vi "Write to Hardware.vi"(8 "error in":errorcluster, 9 "Trigger Values":dbl[](array[numeric]), 10 "Values in":dbl[](array[numeric]), 11 "Address Based Execution Unit Implementation in":refnum<class "Tx Acyclic Execution Unit.lvclass">) -> (0 "error out":errorcluster, 1 "Trigger Values out":dbl[](array[numeric]), 2 "Values out":dbl[](array[numeric]), 3 "Address Based Execution Unit Implementation out":refnum<class "Tx Acyclic Execution Unit.lvclass">)   [LabVIEW 2020, in "AIM MIL-STD-1553 Engine.lvlib" / "Implementation.lvlib" / "Tx Acyclic Execution Unit.lvclass"]
uses:
  Tx Acyclic Execution Unit.lvclass
  Tx Acyclic Execution Unit.lvclass/Tx Acyclic Execution Unit.ctl
  <instrlib>/BTI1553Lib/BTI1553LV.lvlib
  <instrlib>/BTI1553Lib/Private/BC/Data/BC Transmit Acyclic Frame.vi
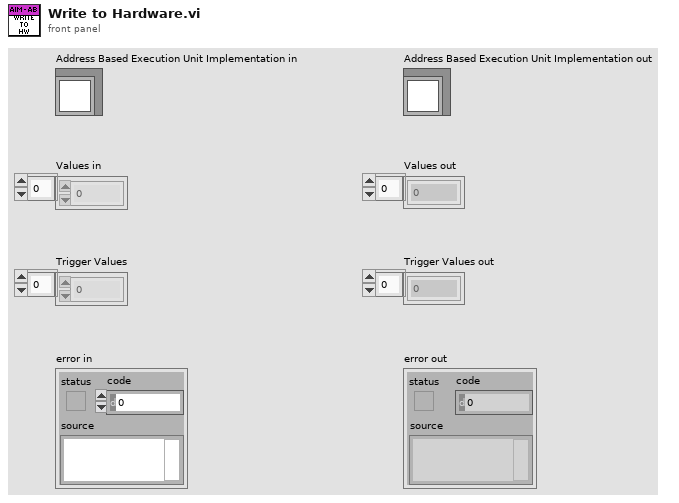
[diagram p1: front panel]
types:
  T1 = typedef "AIM MIL-STD-1553 Engine.lvlib/Implementation.lvlib/Address Based Execution Unit.lvclass/Acyclic Trigger Info.ctl" = cluster{"bus controller handle":u64, "name":string}
  T2 = typedef "AIM MIL-STD-1553 Engine.lvlib/Implementation.lvlib/Address Based Execution Unit.lvclass/Address Write Info.ctl" = cluster{"terminal address":T3, "terminal handle":u64}
  T3 = typedef "Address.ctl" = u16
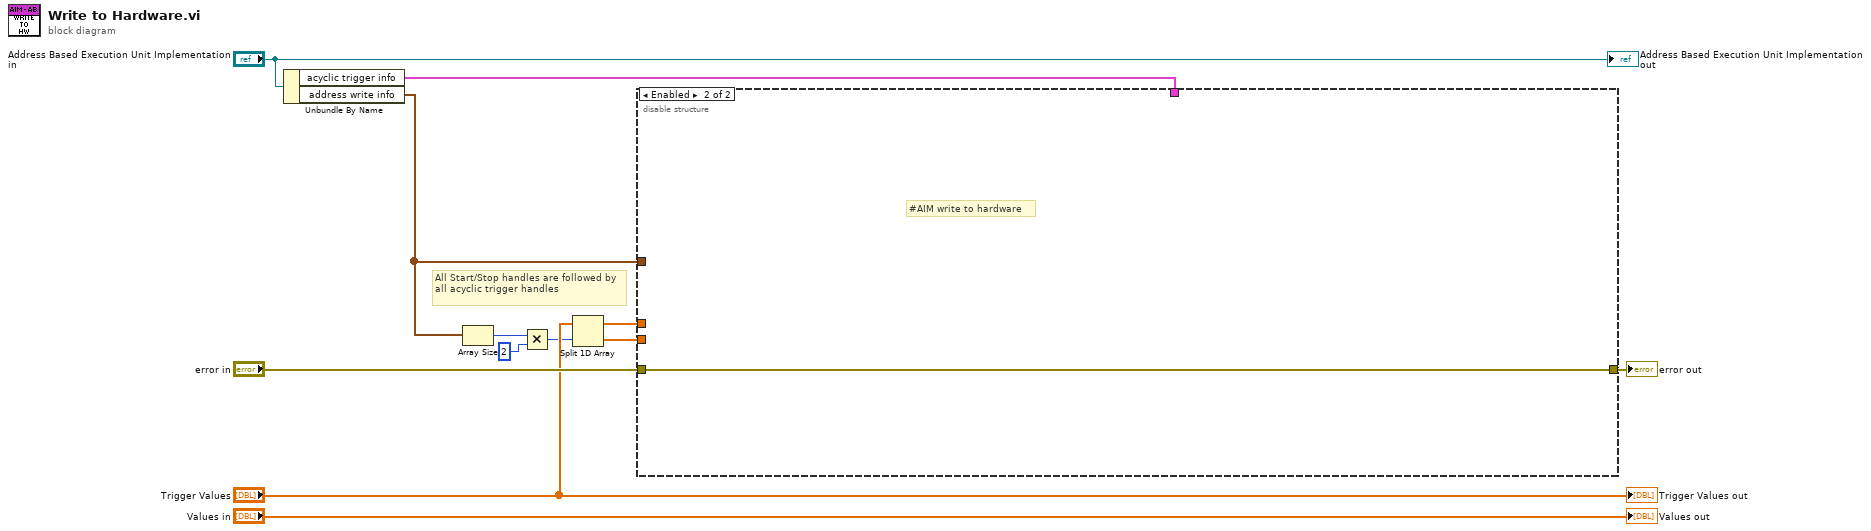
[diagram p0: block diagram]
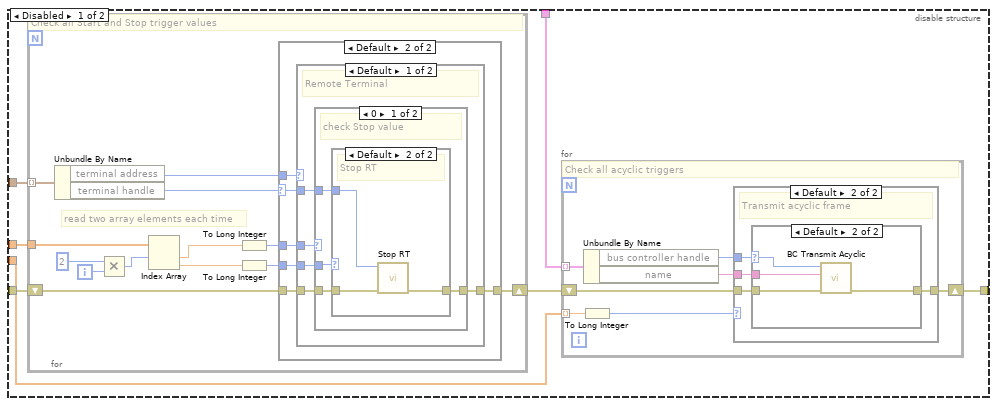
[diagram p2: hidden frame]
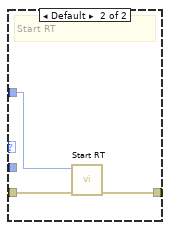
[diagram p7: hidden frame]
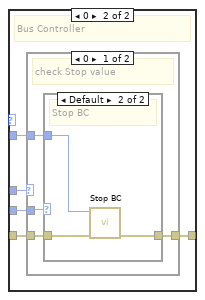
[diagram p8: hidden frame]
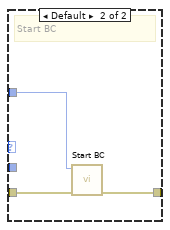
[diagram p10: hidden frame]
diagram:
  # "All Start/Stop handles are followed by all acyclic trigger handles"
  n1 = Unbundle By Name("Address Based Execution Unit Implementation in") -> ("acyclic trigger info"=w1:T1[], "address write info"=w8:T2[])
  n2 = Array Size(array=w8) -> (size(s)=w7:i32)
  n3 = Multiply(x=w7, y=2) -> (x*y=w5:i32)
  n4 = Split 1D Array(array="Trigger Values", index=w5) -> (first subarray=w9:dbl[], second subarray=w2:dbl[])
  n5 = disable-structure shown="Enabled" {
    disable-tunnel: "error in" -> [w19 w89]
    disable-tunnel: w9 -> [w18 _]
    disable-tunnel: w8 -> [w17 _]
    disable-tunnel: [w15 w89] -> w4
    disable-tunnel: w2 -> [w14 _]
    disable-tunnel: w1 -> [w13 _]
    frame Disabled {
      n6 = for {
        tunnel: w17 -> [w49] mode=indexing
        shift-right: [w44] -> w16
        shift-left: w19 -> [w45]
        tunnel: w18 -> [w47]
        i -> [w40]
        # "read two array elements each time"
        # "Check all Start and Stop trigger values"
        n7 = Unbundle By Name(w49) -> ("terminal address"=w48:T3, "terminal handle"=w46:u64)
        n8 = Multiply(x=2, y=w40) -> (x*y=w39:i32)
        n9 = Index Array(array=w47, index #1=w39) -> (element #1=w42:dbl, element #2=w43:dbl)  [unwired: 1 in]
        n10 = To Long Integer(number=w42) -> (32bit integer=w38:i32)
        n11 = To Long Integer(number=w43) -> (32bit integer=w37:i32)
        n12 = case shown="Default" w46 {
          selector: w46 -> [_ w55]
          tunnel: w48 -> [_ w56]
          tunnel: w45 -> [w50 w54]
          tunnel: [w50 w53] -> w44
          tunnel: w38 -> [_ w52]
          tunnel: w37 -> [_ w51]
          frame 0, -1 {
          }
          frame Default {
            n13 = case shown="Default" w56 {
              tunnel: w52 -> [w61 w77]
              tunnel: w51 -> [w57 w73]
              tunnel: w55 -> [w60 w76]
              tunnel: w54 -> [w59 w75]
              tunnel: [w58 w74] -> w53
              frame Default {
                # "Remote Terminal"
                n14 = case shown="0" w61 {
                  tunnel: w60 -> [w63 w71]
                  tunnel: w59 -> [w64 w72]
                  tunnel: [w62 w70] -> w58
                  tunnel: w57 -> [w65 _]
                  frame 0 {
                    # "check Stop value"
                    n15 = case shown="Default" w65 {
                      tunnel: w64 -> [w66 w69]
                      tunnel: w63 -> [_ w68]
                      tunnel: [w66 w67] -> w62
                      frame 0 {
                        # "do nothing"
                      }
                      frame Default {
                        # "Stop RT"
                        n16 = call <instrlib>:"Stop RT.vi"("error in (no error)"=w69, "remote terminal handle in"=w68) -> ("error out"=w67:errorcluster)  [unwired: 8 in, 1 out]
                      }
                    }
                  }
                  frame Default {
                    # "Start RT"
                    n17 = call <instrlib>:"Start RT.vi"("error in (no error)"=w72, "remote terminal handle in"=w71) -> ("error out"=w70:errorcluster)  [unwired: 8 in, 1 out]
                  }
                }
              }
              frame 0 {
                # "Bus Controller"
                n18 = case shown="0" w77 {
                  tunnel: w76 -> [w79 w86]
                  tunnel: w75 -> [w80 w88]
                  tunnel: [w78 w87] -> w74
                  tunnel: w73 -> [w81 _]
                  frame 0 {
                    # "check Stop value"
                    n19 = case shown="Default" w81 {
                      tunnel: w80 -> [w82 w85]
                      tunnel: w79 -> [_ w83]
                      tunnel: [w82 w84] -> w78
                      frame 0 {
                        # "do nothing"
                      }
                      frame Default {
                        # "Stop BC"
                        n20 = call <instrlib>:"Stop BC.vi"("error in (no error)"=w85, "bus controller handle in"=w83) -> ("error out"=w84:errorcluster)  [unwired: 8 in, 1 out]
                      }
                    }
                  }
                  frame Default {
                    # "Start BC"
                    n21 = call <instrlib>:"Start BC.vi"("error in (no error)"=w88, "bus controller handle in"=w86) -> ("error out"=w87:errorcluster)  [unwired: 8 in, 1 out]
                  }
                }
              }
            }
          }
        }
      }
      n22 = for {
        shift-right: [w25] -> w15
        shift-left: w16 -> [w26]
        tunnel: w13 -> [w22] mode=indexing
        tunnel: w14 -> [w24] mode=indexing
        # "Check all acyclic triggers"
        n23 = To Long Integer(number=w24) -> (32bit integer=w23:i32)
        n24 = Unbundle By Name(w22) -> ("bus controller handle"=w21:u64, "name"=w20:string)
        n25 = case shown="Default" w23 {
          tunnel: w26 -> [w27 w30]
          tunnel: [w27 w31] -> w25
          tunnel: w21 -> [_ w29]
          tunnel: w20 -> [_ w28]
          frame 0 {
            # "Do nothing"
          }
          frame Default {
            # "Transmit acyclic frame"
            n26 = case shown="Default" w29 {
              selector: w29 -> [_ w35]
              tunnel: [w32 w36] -> w31
              tunnel: w28 -> [_ w34]
              tunnel: w30 -> [w32 w33]
              frame 0, -1 {
              }
              frame Default {
                n27 = call-poly <instrlib>:"BC Transmit Acyclic.vi"("error in (no error)"=w33, "acyclic frame name"=w34, "bus controller handle in"=w35) -> ("error out"=w36:errorcluster)  [unwired: 7 in, 1 out]
              }
            }
          }
        }
      }
    }
    frame Enabled {
      # "#AIM write to hardware"
    }
  }
  "error out" <- w4
  "Address Based Execution Unit Implementation out" <- "Address Based Execution Unit Implementation in"
  "Values out" <- "Values in"
  "Trigger Values out" <- "Trigger Values"
